vi "write user name.vi"(8 "error in (no error)":errorcluster, 10 "user name":string, 11 "SysCfg Device in":refnum<class "SysCfg Device.lvclass">) -> (0 "error out":errorcluster, 3 "SysCfg Device out":refnum<class "SysCfg Device.lvclass">)   [LabVIEW 2013, in "SMI.lvlib" / "SysCfg Device.lvclass"]
uses:
  SysCfg Device.lvclass
  SysCfg Device.lvclass/SysCfg Device.ctl
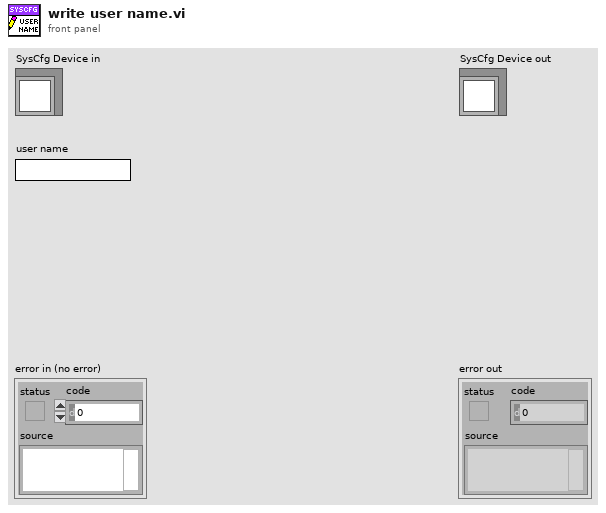
[diagram p1: front panel]
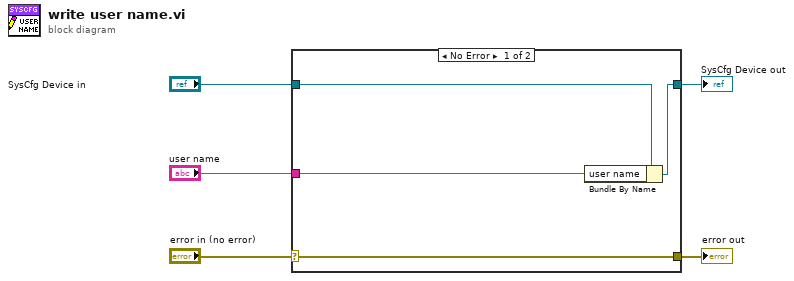
[diagram p0: block diagram]
diagram:
  n1 = case shown="No Error" "error in (no error)" {
    selector: "error in (no error)" -> [w9 w10]
    tunnel: [w9 w10] -> w4
    tunnel: [w7 w11] -> w2
    tunnel: "SysCfg Device in" -> [w8 w11]
    tunnel: "user name" -> [w6 _]
    frame No Error {
      n2 = Bundle By Name(cluster=w8, "user name"=w6) -> (w7:refnum<class "SysCfg Device.lvclass">)
    }
    frame Error {
    }
  }
  "error out" <- w4
  "SysCfg Device out" <- w2
